vi "Programa_robot_final_2.vi"() -> ()   [LabVIEW 2019]
uses:
  <vilib>/Instr/_visa.llb/VISA Configure Serial Port (Instr).vi
  Global_STOP.vi
  <vilib>/regexp/Match Regular Expression.xnode
panel:
  out "return count":u32
  out "lectura puerto serie":u32
  out "dato escrito puerto serie":string
  out "OK, Fault 2":bool
  out "error out":errorcluster {"code" format="%f"}
  in  "STOP TEST 2":bool
  out "Datos_QR 2":string
  out "NUMERO ASICS TESTEADOS":i32
  out "Existe foto anterior?":bool
  out ".not. x?":bool
  in  "Config File":path=path "C:/Trabajo_Robot/Test Asic Javi_2021/Origen Socket SERVO_PCB_BUENO_v5 (muchos asics)/CONFIG/configuracion_robot_CTAV2022A.test"
  in  "SELECCION DE TEST":string(combo)
  in  "?":bool
  out "Boolean":bool
  in  "Cerrar socket":bool
  in  "Abrir socket":bool
  out "Error_QR":bool
  in  "Interruptor Error":bool
  in  "stop socket 2":bool
  out "Bytes at port 3":u32=1
  in  "IN y":string(combo)="00"
  in  "IN x":string(combo)="00"
  in  "NOK y":string(combo)="00"
  in  "NOK x":string(combo)="00"
  in  "OK y":string(combo)="00"
  in  "OK x":string(combo)="00"
  in  "Operator's name":string(combo)="Juan Rodríguez"
  in  "?":bool
  in  "Fichero de registro":path=path "C:/Trabajo_Robot/Pruebas/Pruebas.txt"
  in  "Path Out Report":path=path "C:/Trabajo_Robot/desde Marzo 2023/Pruebas_PC_APD/RESULT_TEST_C_LABP0"
  out "Datos_QR":string
  in  "stop socket":bool
  out "Bytes at port 1":u32
  out "Iteraciones":i32
  out "Lectura buffer":string="1"
  in  "Delay (ms)":dbl=1.0 min=1.0 max=9.0 step=1.0
  out "Bytes at port 2":u32=1
  in  "Interruptor":bool=TRUE
  in  "stop":bool
  # "SI SE PRESIONA EL BOTON STOP PARA DETENER EL TEST,\nHAY QUE APAGAR Y VOLVER A ENCENDER EL ARDUINO"
  # "x: columna en cada bandeja \ny: fila en cada bandeja"
  # "Funcionamiento: en la primera iteración, el efector se desplaza desde el origen hasta la celda\nintroducida, hace una pausa, va a la posición del socket (0,0), hace otra pausa, va a la celda\nde salida y vuelve al origen. En las iteraciones siguientes hará lo mismo pero recorriendo las\nceldas de la bandeja sucesivamente. Que el desplazamiento se produzca hacia una celda de\nla bandeja OK o de la bandeja NOK depende de la salidad del programa de test de Asics."
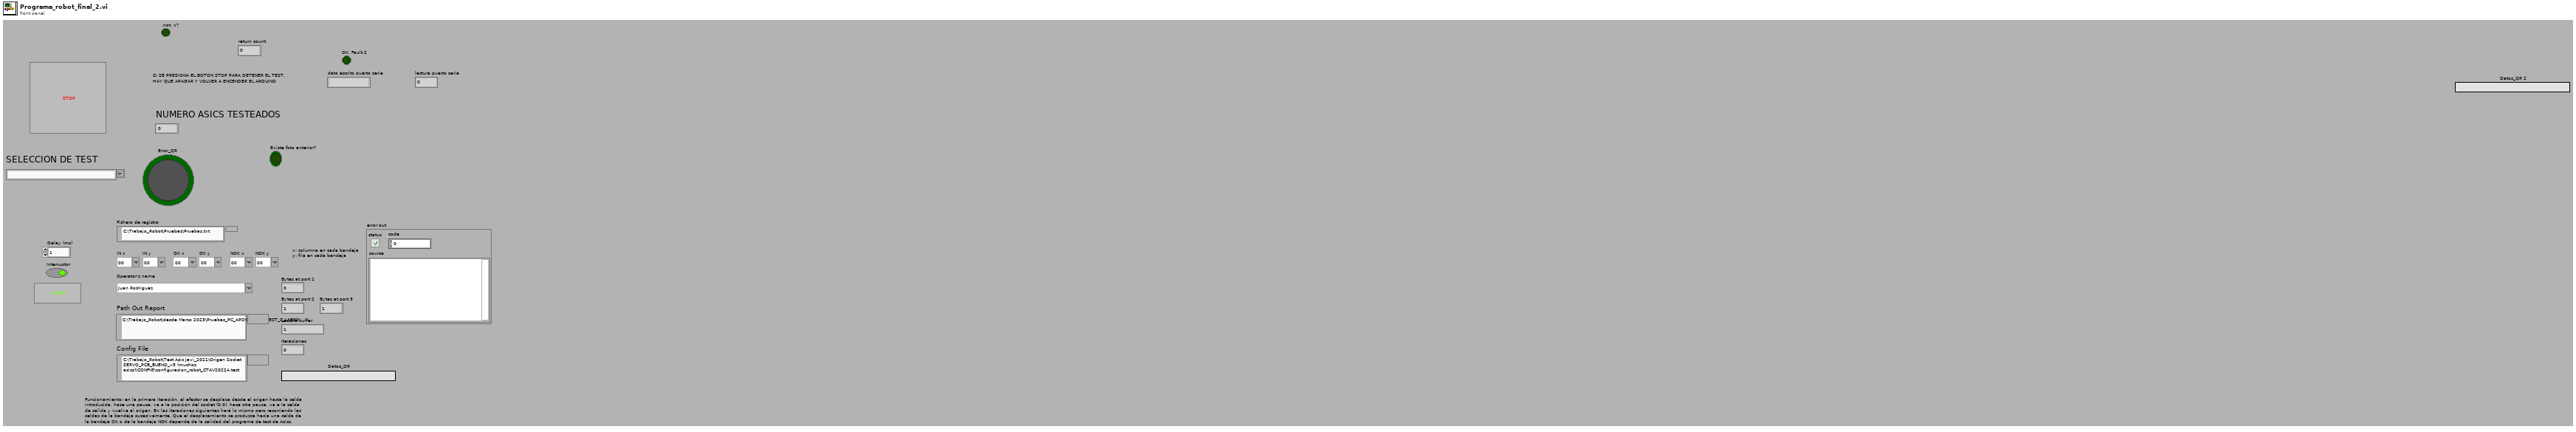
[diagram p1: front panel]
types:
  T1 = enum16{"open", "replace", "create", "open or create", "replace or create", "replace or create with confirmation"}
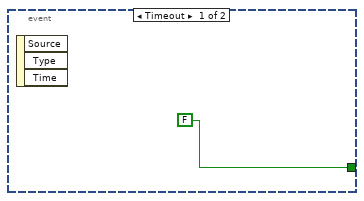
[diagram p2: hidden frame]
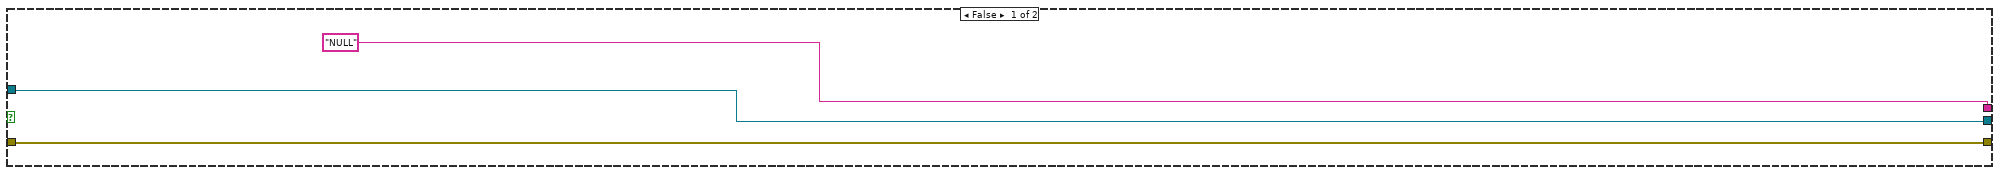
[diagram p5: hidden frame]
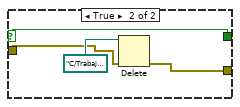
[diagram p8: hidden frame]
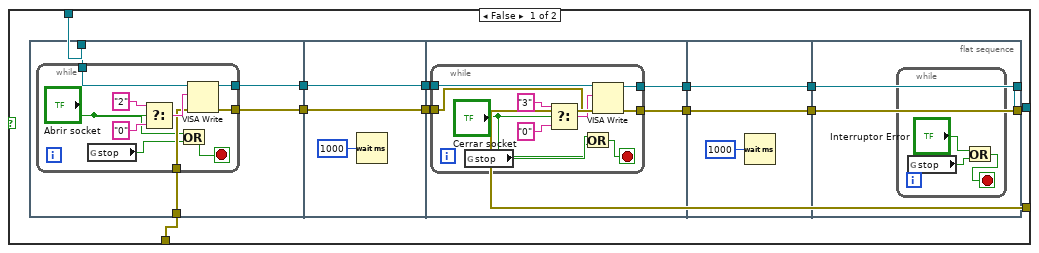
[diagram p9: hidden frame]
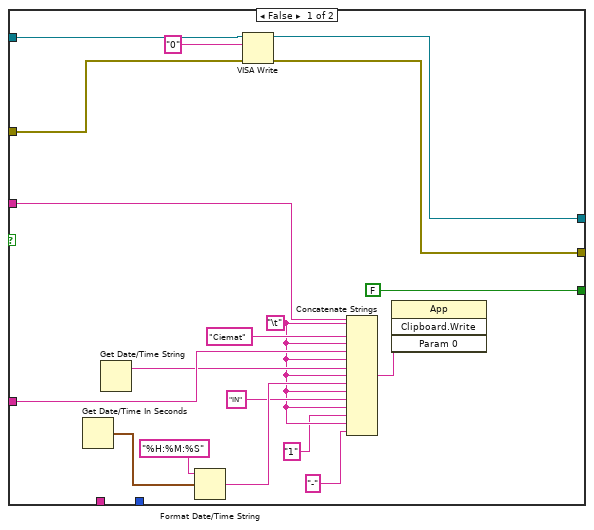
[diagram p10: hidden frame]
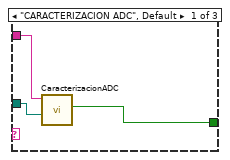
[diagram p11: hidden frame]
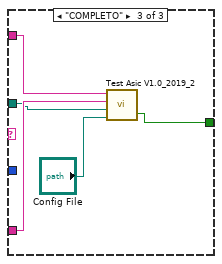
[diagram p12: hidden frame]
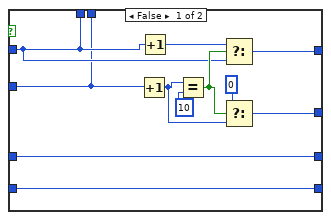
[diagram p14: hidden frame]
diagram:
  n1 = control-ref of="Cerrar socket"() -> (w12:refnum<vi>)
  n2 = control-ref of="stop socket"() -> (w11:refnum<vi>)
  n3 = control-ref of="STOP TEST 2"() -> (w9:refnum<vi>)
  n4 = control-ref of="Abrir socket"() -> (w8:refnum<vi>)
  n5 = control-ref of="stop"() -> (w10:refnum<vi>)
  n6 = control-ref of="Interruptor Error"() -> (w13:refnum<vi>)
  n7 = property class="Bool (strict)"(reference=w9, "Visible"=FALSE) -> ()  [unwired: 1 in, 2 out]
  n8 = property class="Bool (strict)"(reference=w8, "Visible"=FALSE) -> ()  [unwired: 1 in, 2 out]
  n9 = property on="Boolean" class="Bool (strict)"("Visible"=FALSE) -> ()  [unwired: 2 in, 2 out]
  n10 = property class="Bool (strict)"(reference=w13, "Visible"=FALSE) -> ()  [unwired: 1 in, 2 out]
  n11 = property class="Bool (strict)"(reference=w12, "Visible"=FALSE) -> ()  [unwired: 1 in, 2 out]
  n12 = property class="Bool"(reference=w11, "Visible"=FALSE) -> ()  [unwired: 1 in, 2 out]
  n13 = property class="Bool"(reference=w10, "Visible"=FALSE) -> ()  [unwired: 1 in, 2 out]
  n14 = flat-sequence {
    tunnel: [w54] -> w18
    tunnel: ["Fichero de registro"] -> w17
    tunnel: ["SELECCION DE TEST"] -> w16
    tunnel: ["NOK y"] -> w33
    tunnel: ["NOK x"] -> w32
    tunnel: ["OK y"] -> w31
    tunnel: ["OK x"] -> w30
    tunnel: ["IN y"] -> w29
    tunnel: ["IN x"] -> w28
    tunnel: [w57] -> w27
    tunnel: [w58] -> w26
    tunnel: ["IN y"] -> w25
    tunnel: ["IN x"] -> w24
    tunnel: w17 -> [w56]
    frame #0 {
      n15 = while {
        stop <- "?" stop-if-true
        n16 = Not(x="?") -> (.not. x?=w50:bool)
        "Boolean" <- w50
        n17 = property on="Boolean" class="Bool (strict)"("Blinking"=w50) -> ()  [unwired: 2 in, 2 out]
      }
      n18 = global write "Global_STOP.vi" "stop"(FALSE ("stop")) -> ()
    }
    frame #1 {
      n19 = Not(x="?") -> (.not. x?=w54:bool)
      ".not. x?" <- w54
    }
    frame #2 {
      n20 = Open/Create/Replace File(file path (use dialog)=w56, operation (0:open)=T1."open", access (0:read/write)=enum16{"read/write", "read-only", "write-only"}."write-only") -> (refnum out=w69:refnum<file>, error out=w71:errorcluster)  [unwired: 3 in, 1 out]
      n21 = Set File Position(refnum=w69, from (0:start)=enum16{"start", "end", "current"}."end", error in=w71) -> (refnum out=w70:refnum<file>, error out=w72:errorcluster)  [unwired: 1 in]
      n22 = Write to Text File(file (use dialog)=w70, text="\r\n", error in=w72) -> (refnum out=w58:refnum<file>, error out=w57:errorcluster)  [unwired: 1 in, 1 out]
    }
  }
  n23 = Decimal String To Number(string=w25) -> (number=w23:i32)  [unwired: 2 in, 1 out]
  n24 = Decimal String To Number(string=w24) -> (number=w20:i32)  [unwired: 2 in, 1 out]
  n25 = Multiply(x=10, y=w23) -> (x*y=w21:i32)
  n26 = Decimal String To Number(string=w31) -> (number=w35:i32)  [unwired: 2 in, 1 out]
  n27 = Decimal String To Number(string=w30) -> (number=w34:i32)  [unwired: 2 in, 1 out]
  n28 = Decimal String To Number(string=w33) -> (number=w37:i32)  [unwired: 2 in, 1 out]
  n29 = Decimal String To Number(string=w32) -> (number=w36:i32)  [unwired: 2 in, 1 out]
  n30 = call-poly "VISA Configure Serial Port"("VISA resource name"=refnum<visa-resource-name> "COM9", "baud rate (9600)"=u32 9600, "data bits (8)"=u16 8) -> ("VISA resource name out"=w41:refnum<visa-resource-name>, "error out"=w44:errorcluster)  [unwired: 11 in]
  n31 = Add(x=w21, y=w20) -> (x+y=w19:i32)
  n32 = while {
    shift-right: [w82] -> w42
    shift-left: w44 -> [w123]
    tunnel: w41 -> [w121]
    tunnel: [w84] -> w43
    tunnel: w26 -> [w114]
    tunnel: [w113] -> w40
    tunnel: w27 -> [w112]
    tunnel: [w111] -> w39
    tunnel: w28 -> [w109]
    tunnel: w29 -> [w108]
    tunnel: w30 -> [w107]
    tunnel: w31 -> [w106]
    tunnel: w32 -> [w105]
    tunnel: w33 -> [w104]
    shift-right: [w97] -> _
    shift-left: w37 -> [w103]
    shift-right: [w99] -> _
    shift-left: w36 -> [w102]
    shift-right: [w96] -> _
    shift-left: w35 -> [w101]
    shift-right: [w98] -> _
    shift-left: w34 -> [w100]
    tunnel: w19 -> [w95]
    tunnel: w18 -> [w87]
    tunnel: w16 -> [w86]
    tunnel: [w80] -> w14
    i -> [w85]
    stop <- w80 stop-if-true
    n33 = flat-sequence {
      tunnel: w123 -> [w176]
      tunnel: w121 -> [w165]
      tunnel: [w167] -> w120
      tunnel: [w166] -> w119
      tunnel: w109 -> [w146]
      tunnel: w108 -> [w145]
      tunnel: w107 -> [w144]
      tunnel: w106 -> [w143]
      tunnel: w105 -> [w142]
      tunnel: w104 -> [w141]
      tunnel: w120 -> [w913]
      tunnel: w119 -> [w912]
      tunnel: [w911] -> w94
      tunnel: [w910] -> w92
      tunnel: [w909] -> _
      tunnel: w94 -> [w929]
      tunnel: [w927] -> w93
      tunnel: w92 -> [w928]
      tunnel: [w926] -> w91
      tunnel: w93 -> [w949]
      tunnel: w91 -> [w948]
      tunnel: w85 -> [w950]
      tunnel: [w946] -> w90
      tunnel: [w945] -> w89
      tunnel: [w944] -> w88
      tunnel: w85 -> [w1077]
      tunnel: [w1079] -> w117
      tunnel: [w1078] -> w116
      tunnel: [w1075] -> w110
      tunnel: w90 -> [w1074]
      tunnel: w89 -> [w1073]
      tunnel: w88 -> [w1072]
      tunnel: w87 -> [w1067]
      tunnel: w86 -> [w1070]
      tunnel: w85 -> [w1069]
      tunnel: [w1140] -> w115
      tunnel: [w1142] -> w118
      tunnel: w117 -> [w1141]
      tunnel: w116 -> [w1139]
      tunnel: w114 -> [w1146]
      tunnel: [w1145] -> w113
      tunnel: w112 -> [w1144]
      tunnel: [w1143] -> w111
      tunnel: w85 -> [w1136]
      tunnel: w110 -> [w1135]
      tunnel: w103 -> [w1131]
      tunnel: w102 -> [w1134]
      tunnel: w101 -> [w1133]
      tunnel: w100 -> [w1132]
      tunnel: [w1130] -> w97
      tunnel: [w1129] -> w99
      tunnel: [w1128] -> w96
      tunnel: [w1127] -> w98
      tunnel: w95 -> [w1126]
      tunnel: w85 -> [w1125]
      tunnel: [w1124] -> _
      frame #0 {
        n34 = for {
          N: 2 -> [_]
          shift-right: [w788] -> _
          shift-left: w146 -> [w793]
          shift-right: [w791] -> w162
          shift-left: w165 -> [w792]
          shift-right: [w789] -> w161
          shift-left: w176 -> [w790]
          n35 = xnode "Match Regular Expression"("input string"=w793, "regular expression"="-?\\d") -> ("whole match"=w787:string, "after match"=w788:string)  [unwired: 4 in, 3 out]
          n36 = VISA Write(VISA resource name=w792, write buffer=w787, error in (no error)=w790) -> (VISA resource name out=w791:refnum<visa-resource-name>, error out=w789:errorcluster)  [unwired: 1 out]
        }
        n37 = for {
          N: 2 -> [_]
          shift-right: [w666] -> _
          shift-left: w145 -> [w671]
          shift-right: [w669] -> w156
          shift-left: w162 -> [w670]
          shift-right: [w667] -> w155
          shift-left: w161 -> [w668]
          n38 = xnode "Match Regular Expression"("input string"=w671, "regular expression"="-?\\d") -> ("whole match"=w665:string, "after match"=w666:string)  [unwired: 4 in, 3 out]
          n39 = VISA Write(VISA resource name=w670, write buffer=w665, error in (no error)=w668) -> (VISA resource name out=w669:refnum<visa-resource-name>, error out=w667:errorcluster)  [unwired: 1 out]
        }
        n40 = for {
          N: 2 -> [_]
          shift-right: [w544] -> _
          shift-left: w144 -> [w549]
          shift-right: [w547] -> w158
          shift-left: w156 -> [w548]
          shift-right: [w545] -> w157
          shift-left: w155 -> [w546]
          n41 = xnode "Match Regular Expression"("input string"=w549, "regular expression"="-?\\d") -> ("whole match"=w543:string, "after match"=w544:string)  [unwired: 4 in, 3 out]
          n42 = VISA Write(VISA resource name=w548, write buffer=w543, error in (no error)=w546) -> (VISA resource name out=w547:refnum<visa-resource-name>, error out=w545:errorcluster)  [unwired: 1 out]
        }
        n43 = for {
          N: 2 -> [_]
          shift-right: [w422] -> _
          shift-left: w143 -> [w427]
          shift-right: [w425] -> w150
          shift-left: w158 -> [w426]
          shift-right: [w423] -> w149
          shift-left: w157 -> [w424]
          n44 = xnode "Match Regular Expression"("input string"=w427, "regular expression"="-?\\d") -> ("whole match"=w421:string, "after match"=w422:string)  [unwired: 4 in, 3 out]
          n45 = VISA Write(VISA resource name=w426, write buffer=w421, error in (no error)=w424) -> (VISA resource name out=w425:refnum<visa-resource-name>, error out=w423:errorcluster)  [unwired: 1 out]
        }
        n46 = for {
          N: 2 -> [_]
          shift-right: [w300] -> _
          shift-left: w142 -> [w305]
          shift-right: [w303] -> w152
          shift-left: w150 -> [w304]
          shift-right: [w301] -> w151
          shift-left: w149 -> [w302]
          n47 = xnode "Match Regular Expression"("input string"=w305, "regular expression"="-?\\d") -> ("whole match"=w299:string, "after match"=w300:string)  [unwired: 4 in, 3 out]
          n48 = VISA Write(VISA resource name=w304, write buffer=w299, error in (no error)=w302) -> (VISA resource name out=w303:refnum<visa-resource-name>, error out=w301:errorcluster)  [unwired: 1 out]
        }
        n49 = for {
          N: 2 -> [_]
          shift-right: [w178] -> _
          shift-left: w141 -> [w183]
          shift-right: [w181] -> w148
          shift-left: w152 -> [w182]
          shift-right: [w179] -> w147
          shift-left: w151 -> [w180]
          n50 = xnode "Match Regular Expression"("input string"=w183, "regular expression"="-?\\d") -> ("whole match"=w177:string, "after match"=w178:string)  [unwired: 4 in, 3 out]
          n51 = VISA Write(VISA resource name=w182, write buffer=w177, error in (no error)=w180) -> (VISA resource name out=w181:refnum<visa-resource-name>, error out=w179:errorcluster)  [unwired: 1 out]
        }
        n52 = Number To Decimal String(number="Delay (ms)") -> (decimal integer string=w170:string)  [unwired: 1 in]
        n53 = VISA Write(VISA resource name=w148, write buffer=w170, error in (no error)=w147) -> (VISA resource name out=w172:refnum<visa-resource-name>, error out=w171:errorcluster)  [unwired: 1 out]
        n54 = Select(t="1" ("write buffer"), s="Interruptor", f="0" ("write buffer")) -> (s? t:f=w168:string)
        n55 = VISA Write(VISA resource name=w172, write buffer=w168, error in (no error)=w171) -> (VISA resource name out=w167:refnum<visa-resource-name>, error out=w166:errorcluster)  [unwired: 1 out]
      }
      frame #1 {
        n56 = while {
          shift-right: [w919] -> w910
          shift-left: w912 -> [w924]
          tunnel: ["stop socket"] -> _
          shift-right: [w920] -> w911
          shift-left: w913 -> [w925]
          tunnel: ["stop socket"] -> w909
          stop <- w914 stop-if-true
          n57 = property class="Instr"(reference=w925, error in=w924) -> (reference out=w923:refnum<visa-resource-name>, error out=w922:errorcluster, "Bytes at Port"=w921:u32)
          "Bytes at port 1" <- w921
          n58 = VISA Read(VISA resource name=w923, byte count=w921, error in (no error)=w922) -> (VISA resource name out=w920:refnum<visa-resource-name>, read buffer=w918:string, error out=w919:errorcluster)  [unwired: 1 out]
          n59 = Equal?(x="2", y=w918) -> (x = y?=w916:bool)
          n60 = Or(x=w916, y="stop socket") -> (x .or. y?=w914:bool)
        }
      }
      frame #2 {
        n61 = while {
          shift-right: [w935] -> w926
          shift-left: w928 -> [w940]
          tunnel: ["stop socket 2"] -> _
          shift-right: [w936] -> w927
          shift-left: w929 -> [w941]
          tunnel: ["stop socket 2"] -> _
          stop <- w930 stop-if-true
          n62 = property class="Instr"(reference=w941, error in=w940) -> (reference out=w939:refnum<visa-resource-name>, error out=w938:errorcluster, "Bytes at Port"=w937:u32)
          "Bytes at port 3" <- w937
          n63 = VISA Read(VISA resource name=w939, byte count=w937, error in (no error)=w938) -> (VISA resource name out=w936:refnum<visa-resource-name>, read buffer=w934:string, error out=w935:errorcluster)  [unwired: 1 out]
          n64 = Equal?(x="3", y=w934) -> (x = y?=w932:bool)
          n65 = Or(x=w932, y="stop socket 2") -> (x .or. y?=w930:bool)
        }
      }
      frame #3 {
        # "Este bloque realiza la captura y lectura del QR"
        n66 = Greater?(x=w950, y=-1) -> (0:w947:bool)
        n67 = case shown="True" w947 {
          tunnel: [w954 w957] -> w944
          tunnel: w949 -> [w954 w958]
          tunnel: [w953 w956] -> w946
          tunnel: w948 -> [w953 w955]
          tunnel: ["NULL" ("Datos_QR") w959] -> w945
          frame False {
          }
          frame True {
            n68 = while {
              tunnel: [w978] -> w959
              tunnel: w958 -> [w977]
              tunnel: [w973] -> w957
              tunnel: [w972] -> w956
              tunnel: w955 -> [w968]
              stop <- w962 stop-if-true
              n69 = flat-sequence {
                tunnel: w968 -> [w980]
                tunnel: [w981] -> w967
                tunnel: [w994] -> w978
                tunnel: [w992] -> w969
                tunnel: [w991] -> w966
                tunnel: w967 -> [w991]
                frame #0 {
                  # "Éste bloque borra el fichero de imagen\ndel Asic anterior."
                  n70 = call <vilib>:"Check if File or Folder Exists.vi"("error in (no error)"=w980, "path"=path "C:/Trabajo_Robot/Test Asic Javi_2021/Origen Socket SERVO_PCB_BUENO_v5 (muchos asics)/capturaQR.jpg" ("path (use dialog)")) -> ("error out"=w979:errorcluster, "file or folder exists?"=w983:bool, "dup path"=w982:path)  [unwired: 7 in]
                  "Existe foto anterior?" <- w983
                  n71 = case shown="True" w983 {
                    tunnel: w982 -> [w986 w990]
                    tunnel: [w986 w989] -> _
                    tunnel: [w985 w988] -> w981
                    tunnel: w979 -> [w985 w987]
                    frame False {
                    }
                    frame True {
                      n72 = Delete(path (use dialog)=w990, error in=w987) -> (deleted path=w989:path, error out=w988:errorcluster)  [unwired: 3 in, 1 out]
                    }
                  }
                }
                frame #1 {
                  # "Éste bloque realiza la captura de imagen\ndel QR del asic para leer el código."
                  n73 = for {
                    N: 5 -> [_]
                    tunnel: [w999] -> w994
                    tunnel: [w997] -> w992
                    stop <- w995 stop-if-true
                    n74 = call "CapturaImagenyQR_subVI.vi"() -> ("Datos_QR"=w999:string)  [unwired: 11 in]
                    "Datos_QR" <- w999
                    n75 = Equal?(x=w999, y="" ("Datos_QR")) -> (x = y?=w998:bool)
                    n76 = global read "Global_STOP.vi" "stop"() -> (w996:bool)
                    n77 = Not(x=w998) -> (.not. x?=w997:bool)
                    n78 = Compound Arithmetic op=OR(w997, w996) -> (w995:bool)
                  }
                }
              }
              n79 = case shown="False" w969 {
                selector: w969 -> [w1002 w1010]
                tunnel: [w1002 w1010] -> w964
                tunnel: w966 -> [w1004 w1008]
                tunnel: [w1003 w1007] -> w965
                frame False {
                  n80 = Boolean To (0,1)(Boolean=w1002) -> (0, 1=w1005:i16)
                  n81 = call <vilib>:"Error Cluster From Error Code.vi"("error in (no error)"=w1004, "error message (\"\")"="Error de lectura de QR.\nPresione STOP" ("error message (\"\")"), "error code (0)"=w1005) -> ("error out"=w1006:errorcluster)  [unwired: 6 in]
                  n82 = call <vilib>:"Simple Error Handler.vi"("error in (no error)"=w1006) -> ("error out"=w1003:errorcluster)  [unwired: 4 in, 4 out]
                }
                frame True {
                  n83 = Delete(path (use dialog)=path "C:/Trabajo_Robot/Test Asic Javi_2021/Origen Socket SERVO_PCB_BUENO_v5 (muchos asics)/capturaQR.jp", error in=w1008) -> (error out=w1007:errorcluster)  [unwired: 3 in, 2 out]
                }
              }
              n84 = Select(t="1" ("write buffer"), s=w964, f="0" ("write buffer")) -> (s? t:f=w974:string)
              n85 = Not(x=w964) -> (.not. x?=w963:bool)
              "Error_QR" <- w963
              n86 = VISA Write(VISA resource name=w977, write buffer=w974, error in (no error)=w965) -> (VISA resource name out=w971:refnum<visa-resource-name>, error out=w970:errorcluster)  [unwired: 1 out]
              n87 = case shown="True" w964 {
                tunnel: w971 -> [w1022 w1063]
                tunnel: w970 -> [w1021 w1062]
                tunnel: [w1020 w1063] -> w973
                tunnel: [w1019 w1062] -> w972
                frame False {
                  n88 = flat-sequence {
                    tunnel: w1022 -> [w1026]
                    tunnel: [w1025] -> w1018
                    tunnel: [w1024] -> w1017
                    tunnel: w1021 -> [w1023]
                    tunnel: w1018 -> [w1039]
                    tunnel: [w1039] -> w1016
                    tunnel: w1017 -> [w1038]
                    tunnel: [w1038] -> w1015
                    tunnel: w1016 -> [w1043]
                    tunnel: w1015 -> [w1042]
                    tunnel: [w1041] -> w1014
                    tunnel: [w1040] -> w1013
                    tunnel: w1014 -> [w1056]
                    tunnel: [w1056] -> w1012
                    tunnel: w1013 -> [w1055]
                    tunnel: [w1055] -> w1011
                    tunnel: [w1057] -> w1019
                    tunnel: [w1058] -> w1020
                    tunnel: w1012 -> [w1058]
                    tunnel: w1011 -> [w1057]
                    frame #0 {
                      n89 = while {
                        tunnel: w1026 -> [w1036]
                        tunnel: [w1032] -> w1025
                        tunnel: [w1031] -> w1024
                        tunnel: w1023 -> [w1030]
                        stop <- w1027 stop-if-true
                        n90 = global read "Global_STOP.vi" "stop"() -> (w1028:bool)
                        n91 = Select(t="2" ("write buffer"), s="Abrir socket", f="0" ("write buffer")) -> (s? t:f=w1033:string)
                        n92 = Or(x="Abrir socket", y=w1028) -> (x .or. y?=w1027:bool)
                        n93 = VISA Write(VISA resource name=w1036, write buffer=w1033, error in (no error)=w1030) -> (VISA resource name out=w1032:refnum<visa-resource-name>, error out=w1031:errorcluster)  [unwired: 1 out]
                      }
                    }
                    frame #1 {
                      n94 = Wait (ms)(milliseconds to wait=u32 1000) -> ()  [unwired: 1 out]
                    }
                    frame #2 {
                      n95 = while {
                        tunnel: w1043 -> [w1050]
                        tunnel: w1042 -> [w1049]
                        tunnel: [w1048] -> w1041
                        tunnel: [w1047] -> w1040
                        stop <- w1044 stop-if-true
                        n96 = global read "Global_STOP.vi" "stop"() -> (w1046:bool)
                        n97 = Select(t="3" ("write buffer"), s="Cerrar socket", f="0" ("write buffer")) -> (s? t:f=w1051:string)
                        n98 = Or(x=w1046, y="Cerrar socket") -> (x .or. y?=w1044:bool)
                        n99 = VISA Write(VISA resource name=w1050, write buffer=w1051, error in (no error)=w1049) -> (VISA resource name out=w1048:refnum<visa-resource-name>, error out=w1047:errorcluster)  [unwired: 1 out]
                      }
                    }
                    frame #3 {
                      n100 = Wait (ms)(milliseconds to wait=u32 1000) -> ()  [unwired: 1 out]
                    }
                    frame #4 {
                      n101 = while {
                        stop <- w1059 stop-if-true
                        n102 = global read "Global_STOP.vi" "stop"() -> (w1060:bool)
                        n103 = Or(x="Interruptor Error", y=w1060) -> (x .or. y?=w1059:bool)
                      }
                    }
                  }
                }
                frame True {
                }
              }
              n104 = global read "Global_STOP.vi" "stop"() -> (w961:bool)
              n105 = Or(x=w964, y=w961) -> (x .or. y?=w962:bool)
              n106 = case shown="True" w963 {
                frame False {
                }
                frame True {
                  n107 = call "Send Email"() -> ()  [unwired: 11 in, 1 out]
                }
              }
            }
            n108 = Wait (ms)(milliseconds to wait=u32 10000) -> ()  [unwired: 1 out]
          }
        }
        n109 = control-ref of="STOP TEST 2"() -> (w943:refnum<vi>)
        n110 = property class="Bool (strict)"(reference=w943, "Visible"=TRUE) -> ()  [unwired: 1 in, 2 out]
      }
      frame #4 {
        n111 = global read "Global_STOP.vi" "stop"() -> (w1066:bool)
        n112 = Greater?(x=w1077, y=-1) -> (0:w1068:bool)
        n113 = Not(x=w1066) -> (.not. x?=w1065:bool)
        n114 = Compound Arithmetic op=AND(w1068, w1067, w1065) -> (w1064:bool)
        n115 = case shown="True" w1064 {
          tunnel: w1072 -> [w1095 w1102]
          tunnel: w1074 -> [w1094 w1101]
          tunnel: [w1093 w1100] -> w1079
          tunnel: [w1092 w1099] -> w1078
          tunnel: w1073 -> [w1088 w1109]
          tunnel: [FALSE ("Boolean") w1107] -> w1075
          tunnel: "Operator's name" -> [w1086 w1106]
          tunnel: w1070 -> [_ w1105]
          tunnel: w1069 -> [_ w1104]
          frame False {
            w1082 = "\t"
            n116 = Get Date/Time In Seconds() -> (seconds since 1Jan1904=w1090:timestamp)
            n117 = Get Date/Time String() -> (date string=w1085:string)  [unwired: 3 in, 1 out]
            n118 = Format Date/Time String(time format string (%c)="%H:%M:%S", seconds (now)=w1090) -> (date/time string=w1084:string)  [unwired: 1 in]
            n119 = VISA Write(VISA resource name=w1095, write buffer="0", error in (no error)=w1094) -> (VISA resource name out=w1093:refnum<visa-resource-name>, error out=w1092:errorcluster)  [unwired: 1 out]
            n120 = Concatenate Strings(w1088, w1082, "Ciemat", w1082, w1086, w1082, w1085, w1082, w1084, w1082, "IN", w1082, "1", w1082, "-") -> (w1091:string)
            n121 = invoke class="App" method="Clipboard.Write"("Param 0"=w1091) -> ()  [unwired: 3 in, 4 out]
          }
          frame True {
            # "Test de Asics"
            n122 = case shown="\"SUMAS 3 CANALES\"" w1105 {
              tunnel: w1109 -> [w1114 w1116 w1123]
              tunnel: "Path Out Report" -> [w1113 w1118 w1121]
              tunnel: [w1112 w1117 w1119] -> w1107
              tunnel: w1106 -> [_ _ w1122]
              tunnel: w1104 -> [_ w1115 _]
              frame "CARACTERIZACION ADC", Default {
                n123 = call "CaracterizacionADC.vi"("QR code"=w1114, "Path Out Report"=w1113) -> ("OK/NOK"=w1112:bool)  [unwired: 7 in]
              }
              frame "SUMAS 3 CANALES" {
                n124 = call "Test_Sumadores_Javi.vi"("QR"=w1116, "Path"=w1118, "NUMERO DE PASADA DE TEST"=w1115) -> ("Boolean"=w1117:bool)  [unwired: 8 in]
                "NUMERO ASICS TESTEADOS" <- w1115
              }
              frame "COMPLETO" {
                n125 = call "Test Asic V1.0_2019_2.vi"("Config File"="Config File", "Path Out Report"=w1121, "Operator's Name"=w1122, "ASIC'S Number"=w1123) -> ("OK, Fault 2"=w1119:bool)  [unwired: 1 in]
              }
            }
            "OK, Fault 2" <- w1107
            n126 = Select(t="1" ("write buffer"), s=w1107, f="0" ("write buffer")) -> (s? t:f=w1103:string)
            "dato escrito puerto serie" <- w1103
            n127 = VISA Write(VISA resource name=w1102, write buffer=w1103, error in (no error)=w1101) -> (VISA resource name out=w1100:refnum<visa-resource-name>, return count=→"return count":u32, error out=w1099:errorcluster)
          }
        }
      }
      frame #5 {
        n128 = Greater?(x=w1136, y=-1) -> (0:w1137:bool)
        n129 = case shown="True" w1137 {
          tunnel: w1146 -> [w1152 w1185]
          tunnel: [w1152 w1184] -> w1145
          tunnel: w1144 -> [w1151 w1183]
          tunnel: [w1151 w1182] -> w1143
          tunnel: [w1154 w1181] -> w1142
          tunnel: w1141 -> [w1154 w1181]
          tunnel: [w1153 w1180] -> w1140
          tunnel: w1139 -> [w1153 w1180]
          tunnel: w1135 -> [_ w1178]
          tunnel: w1131 -> [w1150 w1177]
          tunnel: w1134 -> [w1149 w1176]
          tunnel: w1133 -> [w1148 w1175]
          tunnel: w1132 -> [w1147 w1174]
          tunnel: [w1150 w1173] -> w1130
          tunnel: [w1149 w1172] -> w1129
          tunnel: [w1148 w1171] -> w1128
          tunnel: [w1147 w1170] -> w1127
          frame False {
          }
          frame True {
            w1157 = "\t"
            # "Registro de datos en fichero"
            n130 = invoke class="App" method="Clipboard.Read"() -> ("Read Clipbrd"=w1179:string)  [unwired: 3 in, 2 out]
            n131 = case shown="True" w1178 {
              tunnel: w1177 -> [w1188 w1201]
              tunnel: w1176 -> [w1187 w1200]
              tunnel: w1175 -> [w1190 w1198]
              tunnel: w1174 -> [w1189 w1199]
              tunnel: [w1192 w1201] -> w1173
              tunnel: [w1191 w1200] -> w1172
              tunnel: [w1190 w1203] -> w1171
              tunnel: [w1189 w1202] -> w1170
              tunnel: [w1188 w1198] -> w1169
              tunnel: [w1187 w1199] -> w1168
              frame False {
                n132 = Increment(x=w1187) -> (x+1=w1196:i32)
                n133 = Increment(x=w1188) -> (x+1=w1193:i32)
                n134 = Equal?(x=w1196, y=10) -> (x = y?=w1194:bool)
                n135 = Select(t=w1193, s=w1194, f=w1188) -> (s? t:f=w1192:i32)
                n136 = Select(t=0, s=w1194, f=w1196) -> (s? t:f=w1191:i32)
              }
              frame True {
                n137 = Increment(x=w1199) -> (x+1=w1207:i32)
                n138 = Increment(x=w1198) -> (x+1=w1204:i32)
                n139 = Equal?(x=w1207, y=10) -> (x = y?=w1205:bool)
                n140 = Select(t=w1204, s=w1205, f=w1198) -> (s? t:f=w1203:i32)
                n141 = Select(t=0, s=w1205, f=w1207) -> (s? t:f=w1202:i32)
              }
            }
            n142 = Write to Text File(file (use dialog)=w1185, text=w1179, error in=w1183) -> (refnum out=w1166:refnum<file>, error out=w1167:errorcluster)  [unwired: 1 in, 1 out]
            n143 = Number To Decimal String(number=w1169) -> (decimal integer string=w1156:string)  [unwired: 1 in]
            n144 = Number To Decimal String(number=w1168) -> (decimal integer string=w1155:string)  [unwired: 1 in]
            n145 = Write to Text File(file (use dialog)=w1166, text=w1157, error in=w1167) -> (refnum out=w1164:refnum<file>, error out=w1165:errorcluster)  [unwired: 1 in, 1 out]
            n146 = Write to Text File(file (use dialog)=w1164, text=w1156, error in=w1165) -> (refnum out=w1161:refnum<file>, error out=w1160:errorcluster)  [unwired: 1 in, 1 out]
            n147 = Write to Text File(file (use dialog)=w1161, text=w1157, error in=w1160) -> (refnum out=w1159:refnum<file>, error out=w1158:errorcluster)  [unwired: 1 in, 1 out]
            n148 = Write to Text File(file (use dialog)=w1159, text=w1155, error in=w1158) -> (refnum out=w1163:refnum<file>, error out=w1162:errorcluster)  [unwired: 1 in, 1 out]
            n149 = Write to Text File(file (use dialog)=w1163, text="\r\n", error in=w1162) -> (refnum out=w1184:refnum<file>, error out=w1182:errorcluster)  [unwired: 1 in, 1 out]
          }
        }
        n150 = Add(x=w1126, y=w1125) -> (x+y=w1124:i32)
      }
    }
    n151 = while {
      shift-right: [w1216] -> w76
      shift-left: w115 -> [w1222]
      tunnel: ["stop"] -> _
      shift-right: [w1217] -> w84
      shift-left: w118 -> [w1223]
      tunnel: [w1212] -> w122
      stop <- w1210 stop-if-true
      # "1"
      # "Mientras se ejecuta este bucle (la espera a que\nArduino termine una iteración), cambiamos los\ndatos de los controladores."
      n152 = property class="Instr"(reference=w1223, error in=w1222) -> (reference out=w1220:refnum<visa-resource-name>, error out=w1219:errorcluster, "Bytes at Port"=w1218:u32)
      "Bytes at port 2" <- w1218
      n153 = VISA Read(VISA resource name=w1220, byte count=w1218, error in (no error)=w1219) -> (VISA resource name out=w1217:refnum<visa-resource-name>, read buffer=w1212:string, return count=w1215:u32, error out=w1216:errorcluster)
      "lectura puerto serie" <- w1215
      n154 = Greater Or Equal?(x=w1215, y=u32 1) -> (x >= y?=w1213:bool)
      n155 = global read "Global_STOP.vi" "stop"() -> (w1209:bool)
      n156 = Or(x=w1213, y="stop") -> (x .or. y?=w1211:bool)
      n157 = Compound Arithmetic op=OR(w1211, w1209) -> (w1210:bool)
    }
    "Lectura buffer" <- w122
    n158 = flat-sequence {
      tunnel: w76 -> [w125]
      tunnel: [w125] -> w75
      tunnel: [w124] -> w73
      frame #0 {
        n159 = global read "Global_STOP.vi" "stop"() -> (w124:bool)
      }
    }
    n160 = case shown="False" w73 {
      selector: w73 -> [_ w135]
      tunnel: [w129 _] -> w81
      tunnel: [w126 w135] -> w77
      tunnel: w75 -> [w127 w134]
      tunnel: [w127 w134] -> w74
      frame False {
        n161 = for {
          N: 3 -> [_]
          tunnel: [w132] -> _
          tunnel: [w130] -> w129
          tunnel: [w130] -> w126
          stop <- w130 stop-if-true
          n162 = call "CapturaImagenyQR_subVI.vi"() -> ("Datos_QR"=w132:string)  [unwired: 11 in]
          "Datos_QR 2" <- w132
          n163 = Equal?(x=w132, y="" ("Datos_QR")) -> (x = y?=w131:bool)
          n164 = Not(x=w131) -> (.not. x?=w130:bool)
        }
      }
      frame True {
      }
    }
    n165 = flat-sequence {
      tunnel: [w138] -> w80
      tunnel: w77 -> [w136]
      frame #0 {
        n166 = global read "Global_STOP.vi" "stop"() -> (w137:bool)
        n167 = Or(x=w136, y=w137) -> (x .or. y?=w138:bool)
      }
    }
    n168 = Boolean To (0,1)(Boolean=w81) -> (0, 1=w79:i16)
    n169 = call <vilib>:"Error Cluster From Error Code.vi"("error in (no error)"=w74, "error message (\"\")"="El asic no se ha colocado en la\n    bandeja de salida,se ha quedado\nen el socket posiblemente por una\nmala succión de la ventosa.\nPresione STOP\n" ("error message (\"\")"), "error code (0)"=w79) -> ("error out"=w78:errorcluster)  [unwired: 6 in]
    n170 = call <vilib>:"Simple Error Handler.vi"("error in (no error)"=w78) -> ("error out"=w82:errorcluster)  [unwired: 4 in, 4 out]
    n171 = case shown="True" w81 {
      selector: w81 -> [w139 w140]
      tunnel: [w139 w140] -> _
      frame False {
      }
      frame True {
        n172 = call "Send Email2"() -> ()  [unwired: 11 in, 1 out]
      }
    }
    "Iteraciones" <- w85
  }
  n173 = flat-sequence {
    frame #0 {
      n174 = local write "STOP TEST 2"(FALSE ("STOP TEST 2")) -> ()
    }
    frame #1 {
      n175 = while {
        stop <- w1225 stop-if-true
        n176 = event shown="[1] \"STOP TEST 2\": Value Change" {
          selector: _ -> [_ _]
          dyn-events: _ -> [_ _]
          timeout: _ -> [_ _]
          tunnel: [FALSE "STOP TEST 2"] -> w1225
          event Timeout {
            n177 = event-data() -> ()  [unwired: 1 in, 3 out]
          }
          event "STOP TEST 2": Value Change {
            n178 = event-data() -> ()  [unwired: 1 in, 6 out]
            n179 = global write "Global_STOP.vi" "stop"("STOP TEST 2") -> ()
            n180 = Wait (ms)(milliseconds to wait=u32 100) -> ()  [unwired: 1 out]
          }
        }
      }
    }
  }
  n181 = Close File(refnum=w40, error in=w39) -> (error out=w38:errorcluster)  [unwired: 1 out]
  n182 = Not(x=w14) -> (.not. x?=w15:bool)
  n183 = call <vilib>:"Simple Error Handler.vi"("error in (no error)"=w38) -> ()  [unwired: 4 in, 5 out]
  n184 = global write "Global_STOP.vi" "stop"(w15) -> ()
  n185 = VISA Close(VISA resource name=w43, error in (no error)=w42) -> (error out=→"error out":errorcluster)
